vi "Pulse Attribute, Set MD5.vi"(6 "error in":errorcluster, 9 "waveform":waveform(dbl)={"t0"=timestamp(3472747248.0780005 s since 1904-01-01), "dt"=2e-06, "Y"=[]}) -> (0 "error out":errorcluster, 1 "New MD5":string, 2 "Old MD5":string, 3 "waveform out":waveform(dbl)={"t0"=timestamp(0 s since 1904-01-01), "dt"=nan, "Y"=[]}, 4 "Temp File":path)   [LabVIEW 2010]
doc: "This function calculates the MD5 message-digest of a waveform and stores it as a waveform attribute."
uses:
  <vilib>/Waveform/WDTFileIO.llb/ Write Waveform to File.vi
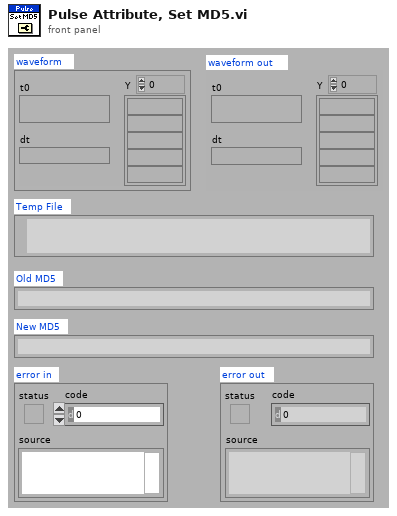
[diagram p1: front panel]
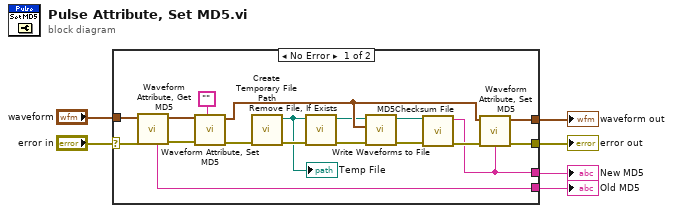
[diagram p0: block diagram]
diagram:
  n1 = case shown="No Error" "error in" {
    selector: "error in" -> [w15 w25]
    tunnel: [w14 w25] -> w5
    tunnel: [w16 _] -> w4
    tunnel: [w17 _] -> w3
    tunnel: "waveform" -> [w13 _]
    tunnel: [w11 _] -> w1
    frame No Error {
      n2 = call "Waveform Attribute, Get MD5.vi"("error in"=w15, "waveform"=w13) -> ("error out"=w19:errorcluster, "waveform dup"=w18:waveform(dbl), "MD5"=w17:string)  [unwired: 5 in]
      n3 = call "Waveform Attribute, Set MD5.vi"("MD5"="", "error in"=w19, "waveform"=w18) -> ("error out"=w22:errorcluster, "waveform out"=w12:waveform(dbl))  [unwired: 5 in]
      n4 = call "Create Temporary File Path.vi"("error in"=w22) -> ("error out"=w10:errorcluster, "filepath"=w8:path)  [unwired: 5 in]
      "Temp File" <- w8
      n5 = call "Remove File, If Exists.vi"("error in"=w10, "filepath"=w8) -> ("error out"=w9:errorcluster, "filepath dup"=w7:path)  [unwired: 4 in]
      n6 = call-poly <vilib>:"Write Waveforms to File.vi"("error in (no error)"=w9, "waveform"=w12, "file path (dialog if empty)"=w7) -> ("error out"=w23:errorcluster, "new file path (Not A Path if cancelled)"=w20:path)  [unwired: 7 in]
      n7 = call <vilib>:"MD5Checksum File.vi"("error in (no error)"=w23, "Path"=w20) -> ("error out"=w24:errorcluster, "MD5 message-digest"=w16:string)  [unwired: 8 in]
      n8 = call "Waveform Attribute, Set MD5.vi"("MD5"=w16, "error in"=w24, "waveform"=w12) -> ("error out"=w14:errorcluster, "waveform out"=w11:waveform(dbl))  [unwired: 5 in]
    }
    frame Error {
    }
  }
  "error out" <- w5
  "New MD5" <- w4
  "Old MD5" <- w3
  "waveform out" <- w1
